vi "Write Active Device.vi"(8 "error in":errorcluster, 10 "Active Device":refnum<vi>, 11 "Instruments in":refnum<class "Instruments.lvclass">) -> (0 "error out":errorcluster, 3 "Instruments out":refnum<class "Instruments.lvclass">)   [LabVIEW 2023, in "Instruments.lvlib" / "Instruments.lvclass"]
uses:
  Library/Instruments.lvclass
  Library/Instruments.lvclass/Instruments.ctl
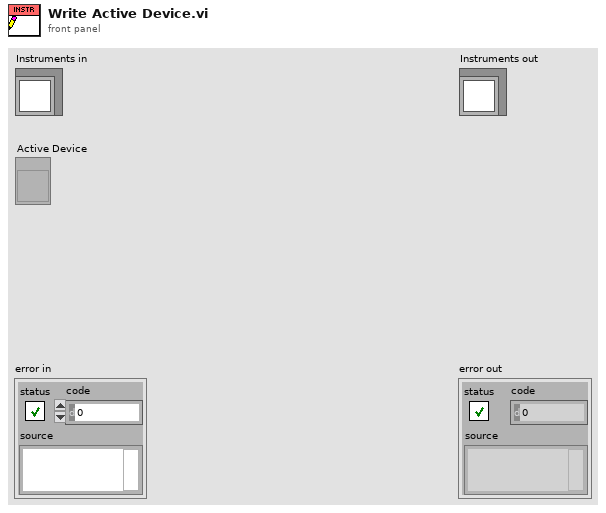
[diagram p1: front panel]
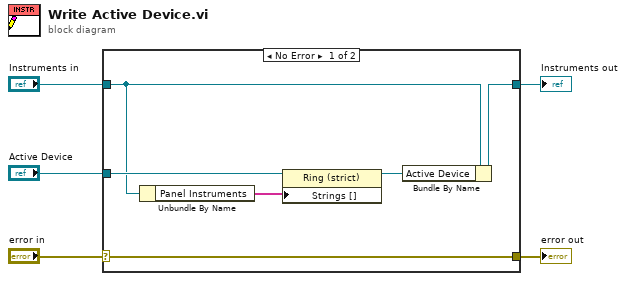
[diagram p0: block diagram]
diagram:
  n1 = case shown="No Error" "error in" {
    selector: "error in" -> [w11 w12]
    tunnel: [w11 w12] -> w4
    tunnel: [w10 w13] -> w2
    tunnel: "Instruments in" -> [w7 w13]
    tunnel: "Active Device" -> [w9 _]
    frame No Error {
      n2 = Unbundle By Name(w7) -> ("Panel Instruments"=w6:string[])
      n3 = property class="Ring (strict)"(reference=w9, "Strings []"=w6) -> (reference out=w8:refnum<vi>)  [unwired: 1 in, 1 out]
      n4 = Bundle By Name(cluster=w7, "Active Device"=w8) -> (w10:refnum<class "Instruments.lvclass">)
    }
    frame Error {
    }
  }
  "error out" <- w4
  "Instruments out" <- w2
